vi "Pretrigger Length - Constant.vi"() -> (3 "Pretrigger length (fraction signal length)":dbl)   [LabVIEW 2020]
doc: "The length of the pretrigger data, recorded and analyzed. Expressed as a fraction of the sample length."
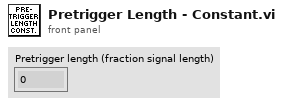
[diagram p1: front panel]
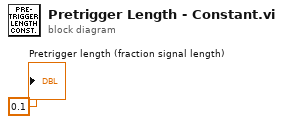
[diagram p0: block diagram]
diagram:
  "Pretrigger length (fraction signal length)" <- 0.1 ("y")
